vi "auto_test.vi"() -> ()   [LabVIEW 2012, in "2013-14.lvrbt"]
uses:
  2013-14.lvrbt
  <vilib>/NXT/Subs/LVHSConnector.ctl
  <vilib>/NXT/LegoClasses/BrickReference/BrickReference.lvclass
  <vilib>/NXT/Block Support/NXT_ButtonSelector.ctl
  E:/FTC/4318/FTC 2013 - 2014/Drivers/AutoDriverControl.ctl
  Drivers/DriveModeControl.ctl
  <vilib>/NXT/Hardware/Plugins/Tetrix DC Motor/TetrixDCMotorAddress.ctl
  <vilib>/NXT/HiTechnic/HiTechnic Controls/HiTechnic Port.ctl
  <vilib>/NXT/Block Support/NXT_InputPort.ctl
  E:/FTC/4318/FTC 2012 - 2013/Controls/SpeedControl.ctl
  <vilib>/NXT/Dual Mode Library/Waits/Wait_Btn_Press.vi
  <vilib>/NXT/NXTIO Xnodes/AddressXNode/NXTIOAddress.xnode
panel:
  in  "Ultra Toggle":bool
  in  "IR Toggle":bool
  in  "NXT In":T1
  out "Distance (cm)":i16
  out "IR Sector":dbl
  out "NXT Out":T1
  # "Just a little tester program that I put together.\nThe two toggle buttons will allow you to\nspecfify if you want to test the IR receiver and\nUltrasonic sensor VIs."
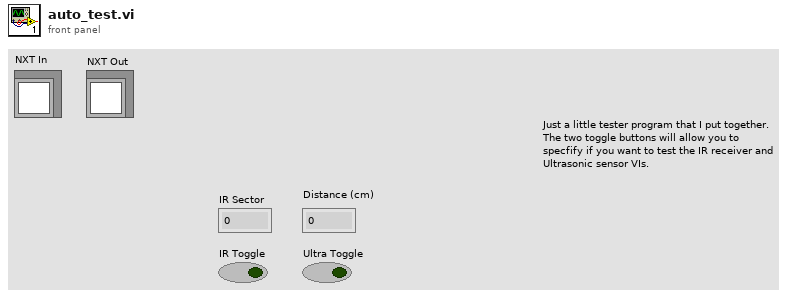
[diagram p1: front panel]
types:
  T1 = typedef "LVHSConnector.ctl" = refnum<class "BrickReference.lvclass">
  T2 = typedef "DriveModeControl.ctl" = enum16{"Drive", "OldManDrive"}
  T3 = typedef "AutoDriverControl.ctl" = enum16{"Init", "Forward", "Reverse", "Left", "Right", "Brake"}
  T4 = typedef "NXT_ButtonSelector.ctl" = u16
  T5 = typedef "HiTechnic Port.ctl" = cluster{"Port":T6, "MUX Port":u8}
  T6 = typedef "NXT_InputPort.ctl" = u8
  T7 = typedef "TetrixDCMotorAddress.ctl" = i16
  T8 = typedef "SpeedControl.ctl" = enum16{"Fast", "Medium", "Slow"}
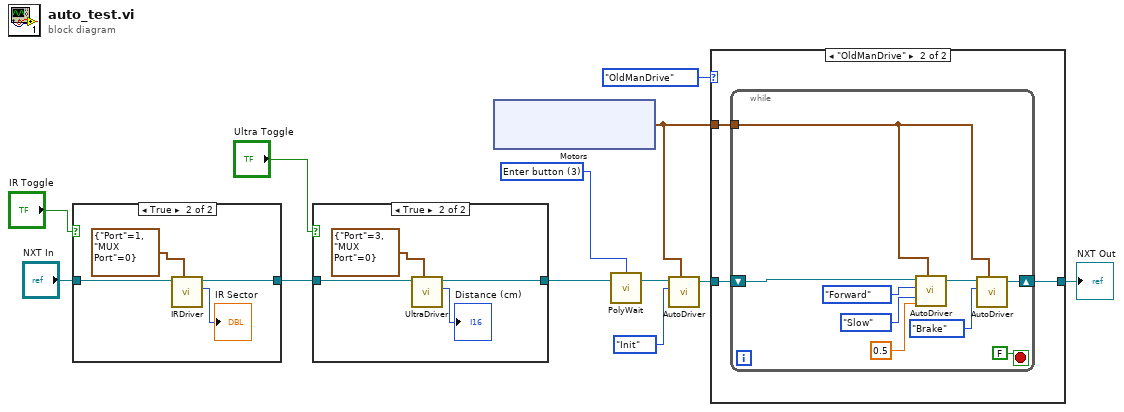
[diagram p0: block diagram]
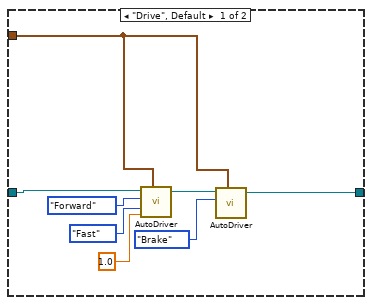
[diagram p2: hidden frame]
diagram:
  w12 = T4 3 items=["Enter button"=3, "Left button"=2, "Right button"=1] ("Button (Enter button)")
  n1 = case shown="True" "IR Toggle" {
    tunnel: [w13 w16] -> w11
    tunnel: "NXT In" -> [w13 w15]
    frame False {
    }
    frame True {
      n2 = call "IRDriver.vi"("Port"=T5 {"Port"=1, "MUX Port"=0}, "NXT In"=w15) -> ("Sector (0-9)"=→"IR Sector":i16, "NXT Out"=w16:T1)  [unwired: 8 in]
    }
  }
  n3 = case shown="True" "Ultra Toggle" {
    tunnel: w11 -> [w18 w21]
    tunnel: [w18 w20] -> w10
    frame False {
    }
    frame True {
      n4 = call "UltraDriver.vi"("Port/MUX"=T5 {"Port"=3, "MUX Port"=0}, "NXT In"=w21) -> ("Distance (cm)"=→"Distance (cm)":i16, "NXT Out"=w20:T1)  [unwired: 8 in]
    }
  }
  n5 = xnode "Motors"() -> ("Motor"=w2:cluster{"TetrixDCMotor":T7, "TetrixDCMotor":T7})
  n6 = call-poly <vilib>:"PolyWait.vi"("NXT"=w10, "Button (Enter button)"=w12) -> ("NXT"=w6:T1)  [unwired: 2 in]
  n7 = call "AutoDriver.vi"("NXT In"=w6, "Motors"=w2, "Direction"=AutoDriverControl."Init") -> ("NXT Out"=w3:T1)  [unwired: 5 in]
  n8 = case shown="\"OldManDrive\"" DriveModeControl."OldManDrive" {
    tunnel: w3 -> [w25 w33]
    tunnel: w2 -> [w24 w32]
    tunnel: [w23 w31] -> w1
    frame "Drive", Default {
      n9 = call "AutoDriver.vi"("NXT In"=w25, "Motors"=w24, "Direction"=AutoDriverControl."Forward", "Speed"=SpeedControl."Fast", "Time (1 sec)"=sgl 1.0) -> ("NXT Out"=w29:T1)  [unwired: 3 in]
      n10 = call "AutoDriver.vi"("NXT In"=w29, "Motors"=w24, "Direction"=AutoDriverControl."Brake") -> ("NXT Out"=w23:T1)  [unwired: 5 in]
    }
    frame "OldManDrive" {
      n11 = while {
        shift-right: [w38] -> w31
        shift-left: w33 -> [w41]
        tunnel: w32 -> [w35]
        stop <- FALSE stop-if-true
        n12 = call "AutoDriver.vi"("NXT In"=w41, "Motors"=w35, "Direction"=AutoDriverControl."Forward", "Speed"=SpeedControl."Slow", "Time (1 sec)"=sgl 0.5) -> ("NXT Out"=w42:T1)  [unwired: 3 in]
        n13 = call "AutoDriver.vi"("NXT In"=w42, "Motors"=w35, "Direction"=AutoDriverControl."Brake") -> ("NXT Out"=w38:T1)  [unwired: 5 in]
      }
    }
  }
  "NXT Out" <- w1
